vi "res_fix_selection.vi"(7 "list":refnum<vi>, 8 "error in":errorcluster) -> (0 "error out":errorcluster, 1 "selected count":i32, 2 "ids of selected":i32[](array[numeric]))   [LabVIEW 2020]
doc: "Fixes selection in result list to valid range."
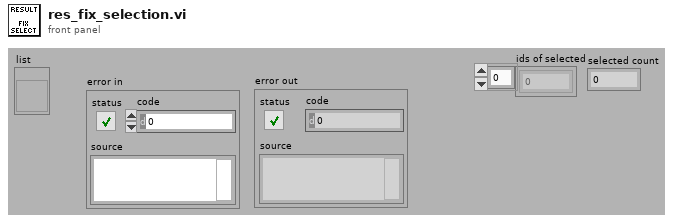
[diagram p1: front panel]
types:
  T1 = typedef "LVRowAndColumnTypeDef.ctl" = cluster{"Row":i32, "Column":i32}
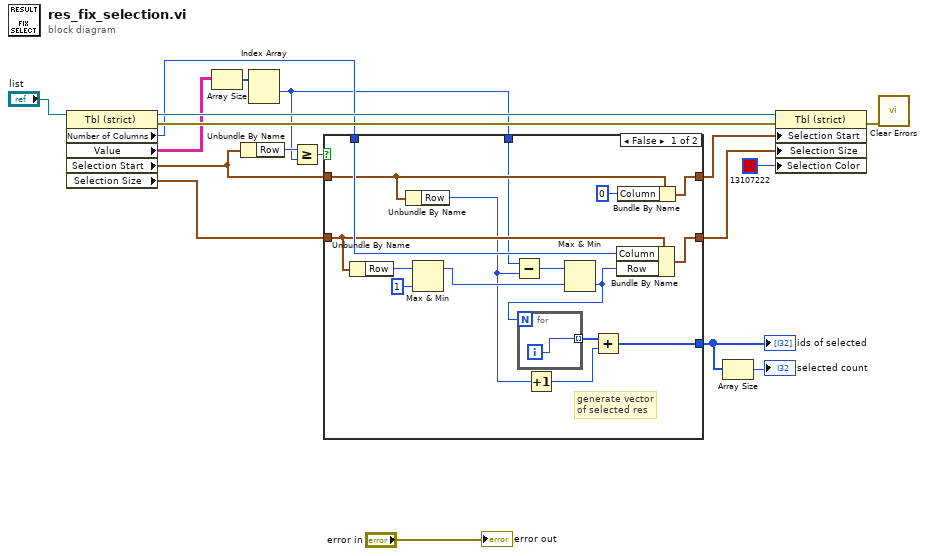
[diagram p0: block diagram]
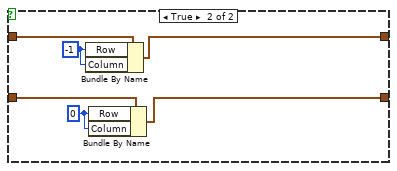
[diagram p2: hidden frame]
diagram:
  n1 = property class="Tbl (strict)"(reference="list") -> (reference out=w15:refnum<vi>, error out=w14:errorcluster, "Number of Columns"=w4:u32, "Value"=w13:string[][], "Selection Start"=w9:T1, "Selection Size"=w8:T1)  [unwired: 1 in]
  n2 = Array Size(array=w13) -> (size(s)=w12:i32[])
  n3 = Unbundle By Name(w9) -> ("Row"=w11:i32)
  n4 = Index Array(array=w12) -> (element #1=w3:i32)  [unwired: 2 in, 1 out]
  n5 = Greater Or Equal?(x=w11, y=w3) -> (x >= y?=w10:bool)
  n6 = case shown="False" w10 {
    tunnel: w9 -> [w27 w41]
    tunnel: [w32 w40] -> w7
    tunnel: w8 -> [w30 w39]
    tunnel: [w34 w37] -> w6
    tunnel: w4 -> [w33 _]
    tunnel: w3 -> [w25 _]
    tunnel: [w20 _] -> w2
    frame False {
      # "generate vector\nof selected res"
      n7 = Unbundle By Name(w30) -> ("Row"=w28:i32)
      n8 = Unbundle By Name(w27) -> ("Row"=w21:i32)
      n9 = Max & Min(x=w28, y=1) -> (max(x,y)=w26:i32)  [unwired: 1 out]
      n10 = Subtract(x=w25, y=w21) -> (x-y=w24:i32)
      n11 = Increment(x=w21) -> (x+1=w19:i32)
      n12 = Max & Min(x=w24, y=w26) -> (min(x,y)=w23:i32)  [unwired: 1 out]
      n13 = for {
        N: w23 -> [_]
        tunnel: [w35] -> w22 mode=indexing
        i -> [w35]
      }
      n14 = Add(x=w22, y=w19) -> (x+y=w20:i32[])
      n15 = Bundle By Name(cluster=w30, "Column"=w33, "Row"=w23) -> (w34:T1)
      n16 = Bundle By Name(cluster=w27, "Column"=0) -> (w32:T1)
    }
    frame True {
      w38 = 0 ("Row")
      w36 = -1 ("Row")
      n17 = Bundle By Name(cluster=w41, "Row"=w36, "Column"=w36) -> (w40:T1)
      n18 = Bundle By Name(cluster=w39, "Row"=w38, "Column"=w38) -> (w37:T1)
    }
  }
  "ids of selected" <- w2
  n19 = Array Size(array=w2) -> (size(s)=→"selected count":i32)
  n20 = property class="Tbl (strict)"(reference=w15, error in=w14, "Selection Start"=w7, "Selection Size"=w6, "Selection Color"=u32 13107222) -> (error out=w17:errorcluster)  [unwired: 1 out]
  n21 = call <vilib>:"Clear Errors.vi"("error in (no error)"=w17) -> ()  [unwired: 5 in, 2 out]
  "error out" <- "error in"
